vi "Citire&Salvare.vi"(9 "NN trained file":path, 11 "Dataset folder":path) -> (0 "Rn output":dbl, 1 "Dataset trained data":path, 2 "Rn input":dbl, 3 "Dataset files":path[][](array[path]), 4 "Nume clase":string[](array[string]))   [LabVIEW 2024]
uses:
  <vilib>/National Instruments/NI Super Simple Neural Networks/Types/1D Array.ctl
  <vilib>/National Instruments/NI Super Simple Neural Networks/Neural Network.lvclass
  <vilib>/National Instruments/NI Super Simple Neural Networks/Types/Teaching Vector.ctl
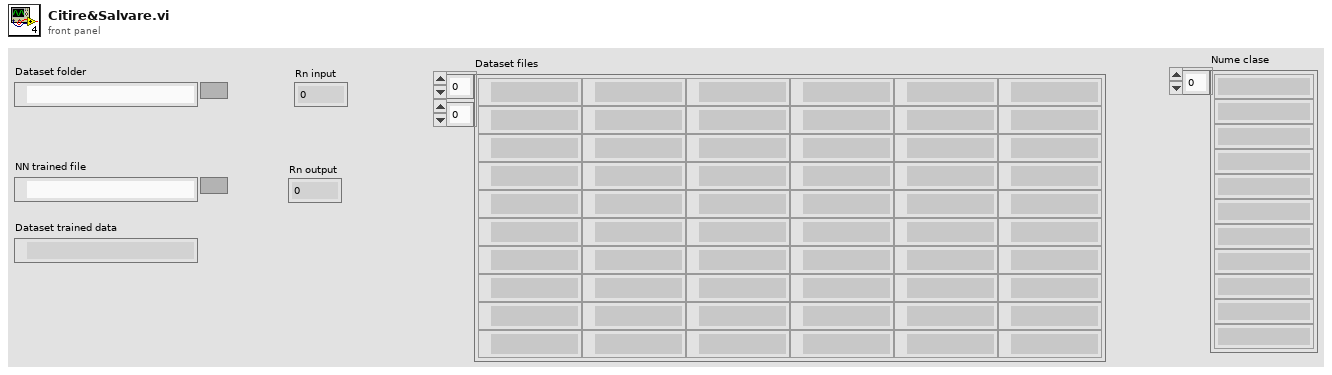
[diagram p1: front panel]
types:
  T1 = enum16{"open", "replace", "create", "open or create", "replace or create", "replace or create with confirmation"}
  T2 = typedef "Neural Network.lvclass/Teaching Vector.ctl" = cluster{"Inputs":T3, "Expected Outputs":T3}
  T3 = typedef "Neural Network.lvclass/1D Array.ctl" = cluster{"1D Array":dbl[]}
  T4 = typedef "imagedata.ctl" = cluster{"image type":i32, "image depth":i32, "image":u8[], "mask":u8[], "colors":u32[], "Rectangle":cluster{"left":i16, "top":i16, "right":i16, "bottom":i16}}
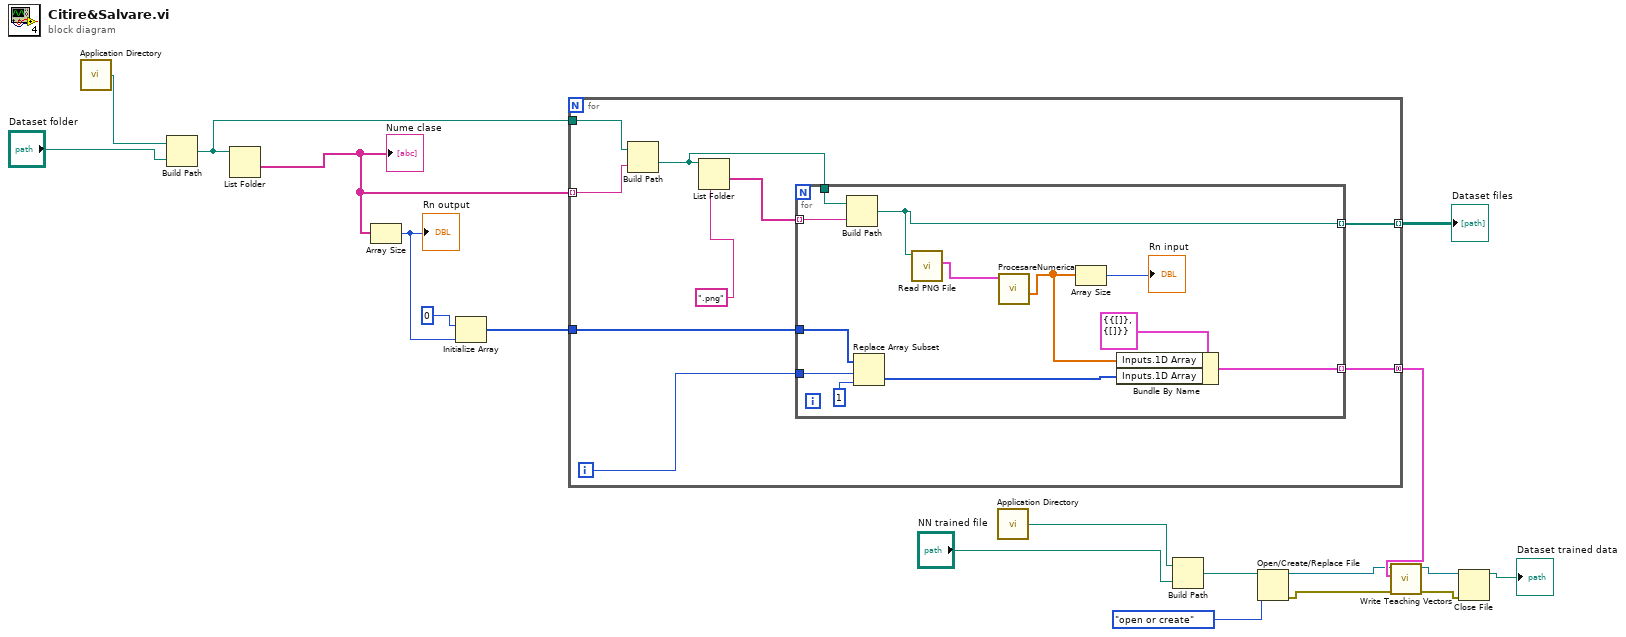
[diagram p0: block diagram]
diagram:
  n1 = call <vilib>:"Application Directory.vi"() -> ("Application Directory"=w18:path)
  n2 = Build Path(base path=w18, name or relative path="Dataset folder") -> (appended path=w14:path)
  n3 = List Folder(path=w14) -> (folder names=w13:string[])  [unwired: 3 in, 3 out]
  "Nume clase" <- w13
  n4 = Array Size(array=w13) -> (size(s)=w15:i32)
  "Rn output" <- w15
  n5 = Initialize Array(0, w15) -> (w12:i32[])
  n6 = for {
    tunnel: w14 -> [w26]
    tunnel: w13 -> [w25] mode=indexing
    tunnel: w12 -> [w22]
    tunnel: [w21] -> w11 mode=indexing
    tunnel: [w20] -> w6 mode=concatenating
    i -> [w23]
    n7 = Build Path(base path=w26, name or relative path=w25) -> (appended path=w24:path)
    n8 = List Folder(path=w24, pattern=".png") -> (folder names=w19:string[])  [unwired: 2 in, 3 out]
    n9 = for {
      tunnel: w24 -> [w39]
      tunnel: w23 -> [w38]
      tunnel: w22 -> [w37]
      tunnel: [w36] -> w21 mode=indexing
      tunnel: [w30] -> w20 mode=indexing
      tunnel: w19 -> [w29] mode=indexing
      n10 = Build Path(base path=w39, name or relative path=w29) -> (appended path=w36:path)
      n11 = Replace Array Subset(array=w37, new element=1, index=w38) -> (w32:i32[])
      n12 = call <vilib>:"Read PNG File.vi"("path to PNG file"=w36) -> ("image data"=w35:T4)  [unwired: 8 in, 2 out]
      n13 = call "ProcesareNumerica.vi"("image data"=w35) -> ("image array"=w31:dbl[])  [unwired: 9 in, 1 out]
      n14 = Array Size(array=w31) -> (size(s)=→"Rn input":i32)
      n15 = Bundle By Name(cluster=T2 {"Inputs"={"1D Array"=[]}, "Expected Outputs"={"1D Array"=[]}} ("Teaching Vector"), "Inputs.1D Array"=w31, "Inputs.1D Array"=w32) -> (w30:T2)
    }
  }
  "Dataset files" <- w11
  n16 = call <vilib>:"Application Directory.vi"() -> ("Application Directory"=w9:path)
  n17 = Build Path(base path=w9, name or relative path="NN trained file") -> (appended path=w8:path)
  n18 = Open/Create/Replace File(file path (use dialog)=w8, operation (0:open)=T1."open or create") -> (refnum out=w4:refnum<file>, error out=w5:errorcluster)  [unwired: 4 in, 1 out]
  n19 = call <vilib>:"Write Teaching Vectors.vi"("Error In"=w5, "Teaching Vectors"=w6, "Teaching File Ref In"=w4) -> ("Error Out"=w1:errorcluster, "Teaching File Ref Out"=w3:refnum<file>)  [unwired: 7 in]
  n20 = Close File(refnum=w3, error in=w1) -> (path=→"Dataset trained data":path)  [unwired: 1 out]
